vi "CRYGet Channel From Signal Type.vi"(8 "Calibration":T1 {"Calibration 2D"."Sens Curve"."Z data" items=["dB", "Lin"]; "Calibration 2D"."Sens Curve"."X data" items=["dB", "Lin"]; "Calibration 2D"."Sens Curve"."Y data" items=["dB", "Lin"]; "Calibration 2D"."Sens Curve"."Z dB ref" format="%.1f"; "Calibration 2D"."Sens Curve"."Z axis" items=["Log", "Lin"]; "Calibration 2D"."Sens Curve"."X dB ref" format="%.1f"; "Calibration 2D"."Sens Curve"."X axis" items=["Log", "Lin"]; "Calibration 2D"."Sens Curve"."Y axis" items=["Log", "Lin"]; "Calibration 2D"."Sens Curve"."Y dB ref" format="%.1f"; "Calibration 2D"."Sens Curve"."Curve"."z" format="%.2f"; "Calibration 2D"."Sens Curve"."Curve"."y" format="%.2f"; "Calibration 2D"."Sens Curve"."Curve"."x" format="%.2f"; "Calibration 2D"."EQ Curve"."Z data" items=["dB", "Lin"]; "Calibration 2D"."EQ Curve"."X data" items=["dB", "Lin"]; "Calibration 2D"."EQ Curve"."Y data" items=["dB", "Lin"]; "Calibration 2D"."EQ Curve"."Z dB ref" format="%.1f"; "Calibration 2D"."EQ Curve"."Z axis" items=["Log", "Lin"]; "Calibration 2D"."EQ Curve"."X dB ref" format="%.1f"; "Calibration 2D"."EQ Curve"."X axis" items=["Log", "Lin"]; "Calibration 2D"."EQ Curve"."Y axis" items=["Log", "Lin"]; "Calibration 2D"."EQ Curve"."Y dB ref" format="%.1f"; "Calibration 2D"."EQ Curve"."Curve"."z" format="%.2f"; "Calibration 2D"."EQ Curve"."Curve"."y" format="%.2f"; "Calibration 2D"."EQ Curve"."Curve"."x" format="%.2f"; "Calibration 2D"."Corr Curve"."Z data" items=["dB", "Lin"]; "Calibration 2D"."Corr Curve"."X data" items=["dB", "Lin"]; "Calibration 2D"."Corr Curve"."Y data" items=["dB", "Lin"]; "Calibration 2D"."Corr Curve"."Z dB ref" format="%.1f"; "Calibration 2D"."Corr Curve"."Z axis" items=["Log", "Lin"]; "Calibration 2D"."Corr Curve"."X dB ref" format="%.1f"; "Calibration 2D"."Corr Curve"."X axis" items=["Log", "Lin"]; "Calibration 2D"."Corr Curve"."Y axis" items=["Log", "Lin"]; "Calibration 2D"."Corr Curve"."Y dB ref" format="%.1f"; "Calibration 2D"."Corr Curve"."Curve"."z" format="%.2f"; "Calibration 2D"."Corr Curve"."Curve"."y" format="%.2f"; "Calibration 2D"."Corr Curve"."Curve"."x" format="%.2f"; "Calibration 2D"."Calibration"."EQ Step size" items=["R10", "R20", "R40", "R80", "User"]; "Calibration 2D"."Calibration"."Corr Step size" items=["R10", "R20", "R40", "R80", "User"]}, 10 "Signal Type Name Array In":string[](array[string]), 11 "In/Out?":bool) -> (2 "equal Index Out":i32[](array[numeric]), 3 "Channel Name Array Out":string[](array[string]))   [LabVIEW 2013]
uses:
  Typedef Control/CRYCalibration All Cluster.ctl
  Typedef Control/CRYCalibration 2DCluster.ctl
  Typedef Control/CRYCalibration Cluster.ctl
  Typedef Control/CRYData Cluster.ctl
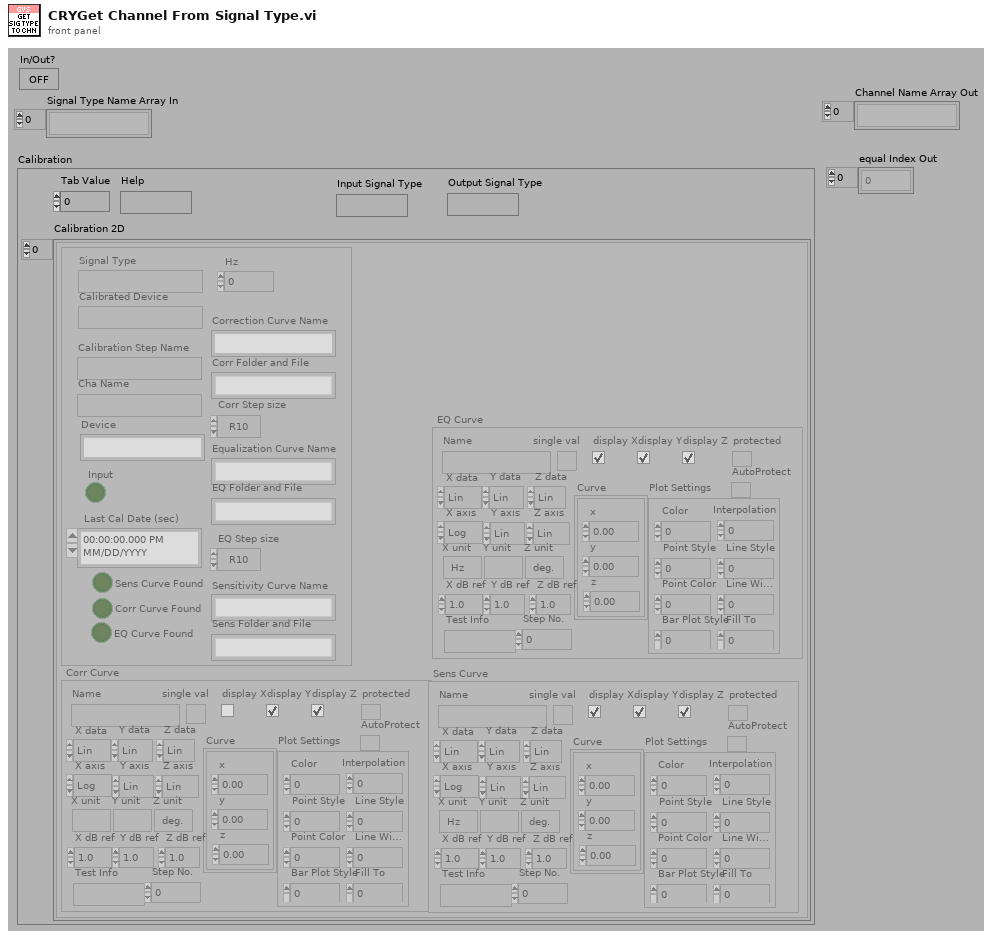
[diagram p1: front panel]
types:
  T1 = typedef "CRYCalibration All Cluster.ctl" = cluster{"Calibration 2D":T2[], "Help":string, "Tab Value":i32, "Input Signal Type":string, "Output Signal Type":string}
  T2 = typedef "CRYCalibration 2DCluster.ctl" = cluster{"Calibration":T3, "Corr Curve":T4, "EQ Curve":T4, "Sens Curve":T4}
  T3 = typedef "CRYCalibration Cluster.ctl" = cluster{"Calibration Step Name":string, "Device":string, "Correction Curve Name":string, "Equalization Curve Name":string, "Sensitivity Curve Name":string, "Corr Folder and File":string, "EQ Folder and File":string, "Sens Folder and File":string, "Corr Step size":u16, "EQ Step size":u16, "Input":bool, "Last Cal Date (sec)":timestamp, "Cha Name":string, "Corr Curve Found":bool, "EQ Curve Found":bool, "Sens Curve Found":bool, "Signal Type":string, "Calibrated Device":string, "Hz":u32}
  T4 = typedef "CRYData Cluster.ctl" = cluster{"Name":string, "Curve":cluster{"x":dbl, "y":dbl, "z":dbl}[], "X data":u16, "Y data":u16, "Z data":u16, "X axis":u16, "Y axis":u16, "Z axis":u16, "X unit":string, "Y unit":string, "Z unit":string, "X dB ref":dbl, "Y dB ref":dbl, "Z dB ref":dbl, "single val":bool, "protected":bool, "display X":bool, "display Y":bool, "display Z":bool, "Test Info":string, "Step No.":i32, "Plot Settings":cluster{"Color":u32, "Interpolation":u8, "Point Style":u8, "Line Style":u8, "Point Color":u32, "Line Width":u8, "Bar Plot Style":u8, "Fill To":i16}, "AutoProtect":bool}
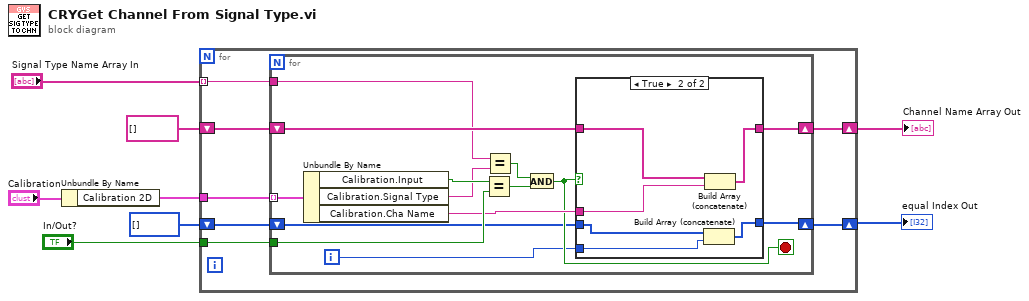
[diagram p0: block diagram]
diagram:
  n1 = Unbundle By Name("Calibration") -> ("Calibration 2D"=w7:T2[])
  n2 = for {
    tunnel: w7 -> [w15]
    shift-right: [w13] -> w6
    shift-left: string[] [] -> [w14]
    tunnel: "Signal Type Name Array In" -> [w11] mode=indexing
    tunnel: "In/Out?" -> [w12]
    shift-right: [w10] -> w2
    shift-left: i32[] [] ("Array") -> [w9]
    n3 = for {
      tunnel: w15 -> [w29] mode=indexing
      tunnel: w12 -> [w25]
      tunnel: w11 -> [w23]
      shift-right: [w27] -> w13
      shift-left: w14 -> [w28]
      shift-right: [w17] -> w10
      shift-left: w9 -> [w16]
      i -> [w18]
      stop <- w19 stop-if-true
      n4 = Unbundle By Name(w29) -> ("Calibration.Input"=w26:bool, "Calibration.Signal Type"=w24:string, "Calibration.Cha Name"=w20:string)
      n5 = Equal?(x=w26, y=w25) -> (x = y?=w21:bool)
      n6 = Equal?(x=w23, y=w24) -> (x = y?=w22:bool)
      n7 = And(x=w22, y=w21) -> (x .and. y?=w19:bool)
      n8 = case shown="True" w19 {
        tunnel: w28 -> [w31 w35]
        tunnel: [w31 w36] -> w27
        tunnel: w20 -> [_ w37]
        tunnel: w18 -> [_ w33]
        tunnel: [w30 w32] -> w17
        tunnel: w16 -> [w30 w34]
        frame False {
        }
        frame True {
          n9 = Build Array (concatenate)(w34, w33) -> (w32:i32[])
          n10 = Build Array (concatenate)(w35, w37) -> (w36:string[])
        }
      }
    }
  }
  "Channel Name Array Out" <- w6
  "equal Index Out" <- w2
